vi "Strings und Zeitstempel verknuepfen neu.vi"(5 "LF 1 -2":bool, 7 "aufsteigend":bool, 8 "String 2 hinzufügen":string, 9 "String 1 hinzufügen":string, 11 "Eingangs String":string) -> (2 "Verknüpfter String":string)   [LabVIEW 2020, in "allgemeine Sub-VIs.lvlib"]
uses:
  allgemeine Sub-VIs.lvlib
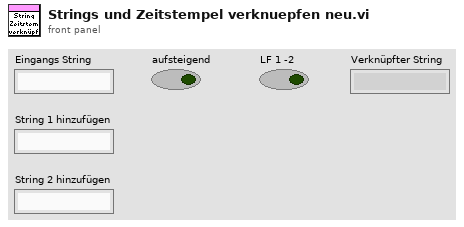
[diagram p1: front panel]
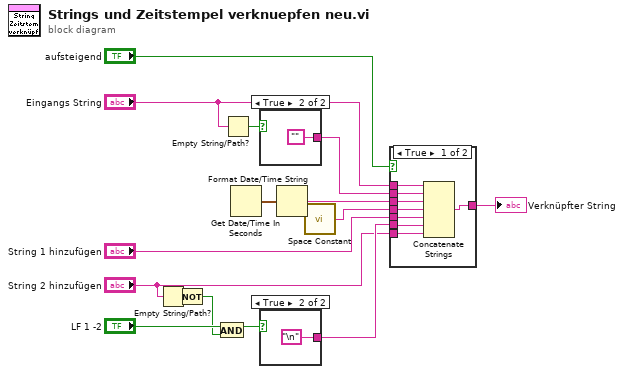
[diagram p0: block diagram]
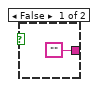
[diagram p2: hidden frame]
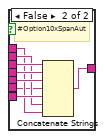
[diagram p3: hidden frame]
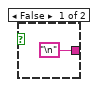
[diagram p4: hidden frame]
diagram:
  n1 = Empty String/Path?(string/path="String 2 hinzufügen") -> (empty?=w2:bool)
  n2 = Not(x=w2) -> (.not. x?=w1:bool)
  n3 = And(x="LF 1 -2", y=w1) -> (x .and. y?=w4:bool)
  n4 = Empty String/Path?(string/path="Eingangs String") -> (empty?=w7:bool)
  n5 = Get Date/Time In Seconds() -> (seconds since 1Jan1904=w13:timestamp)
  n6 = case shown="True" w7 {
    tunnel: ["\n" ""] -> w14
    frame False {
    }
    frame True {
    }
  }
  n7 = case shown="True" w4 {
    tunnel: ["" "\n"] -> w5
    frame False {
    }
    frame True {
    }
  }
  n8 = Format Date/Time String(seconds (now)=w13) -> (date/time string=w12:string)  [unwired: 2 in]
  n9 = call <vilib>:"Space Constant.vi"() -> ("String"=w11:string)
  n10 = case shown="True" "aufsteigend" {
    tunnel: "Eingangs String" -> [w27 w29]
    tunnel: w14 -> [w26 w30]
    tunnel: w12 -> [w25 w35]
    tunnel: w11 -> [w24 w34]
    tunnel: "String 1 hinzufügen" -> [w23 w33]
    tunnel: "String 2 hinzufügen" -> [w21 w32]
    tunnel: [w22 w31] -> w9
    tunnel: w5 -> [w20 w28]
    frame True {
      n11 = Concatenate Strings(w27, w26, w25, w24, w23, w20, w21) -> (w22:string)
    }
    frame False {
      # "#Option10xSpanAut"
      n12 = Concatenate Strings(w35, w34, w33, w28, w32, w30, w29) -> (w31:string)
    }
  }
  "Verknüpfter String" <- w9
